vi "experiment_med_read_FF.vi"() -> ()   [LabVIEW 2018]
uses:
  FPGA/Feed forward/FeedForwardState.ctl
  <vilib>/rvi/Emulation/niFpgaSctlEmulationGetInTimedLoop.vi
  <vilib>/rvi/Memory/Memory_Emulation/nirvimemoryFastEmulation.vi
  <vilib>/rvi/Memory/Memory_Emulation/nirvimemoryEmulation.vi
  <vilib>/rvi/Emulation/niFpgaEmulationIsFPGAContextNoSignature.vi
  <vilib>/rvi/DataTransferAndStorage/Container/Common/niFpgaContainerGetUniqueNameForEmu.vi
  <vilib>/rvi/Emulation/niFpgaProcessEmulError.vi
  <vilib>/rvi/errors/nirviReportUnexpectedCaseInternalError (U32).vi
  <instrlib>/_niInstr/Basic Elements/v1/FPGA/Private/Count Down U8.vi
  <vilib>/rvi/DataTransferAndStorage/Container/XNode/niFpgaContainer.xnode
  <instrlib>/_niInstr/Basic Elements/v1/FPGA/niInstr Basic Elements v1 FPGA.lvlib
panel:
  out "Array":dbl[](array[numeric])
  out "Waveform Graph":dbl[](graph)
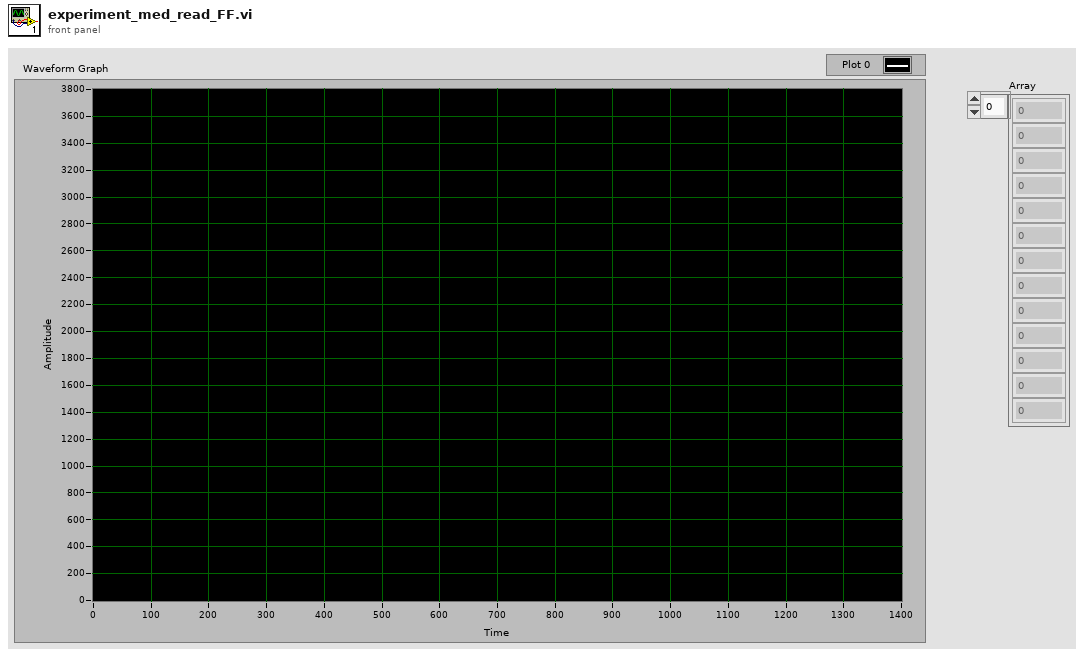
[diagram p1: front panel]
types:
  T1 = typedef "FeedForwardState.ctl" = enum16{"Idle", "Wait for trigger", "Read FF", "Clear FF", "Wait for reset"}
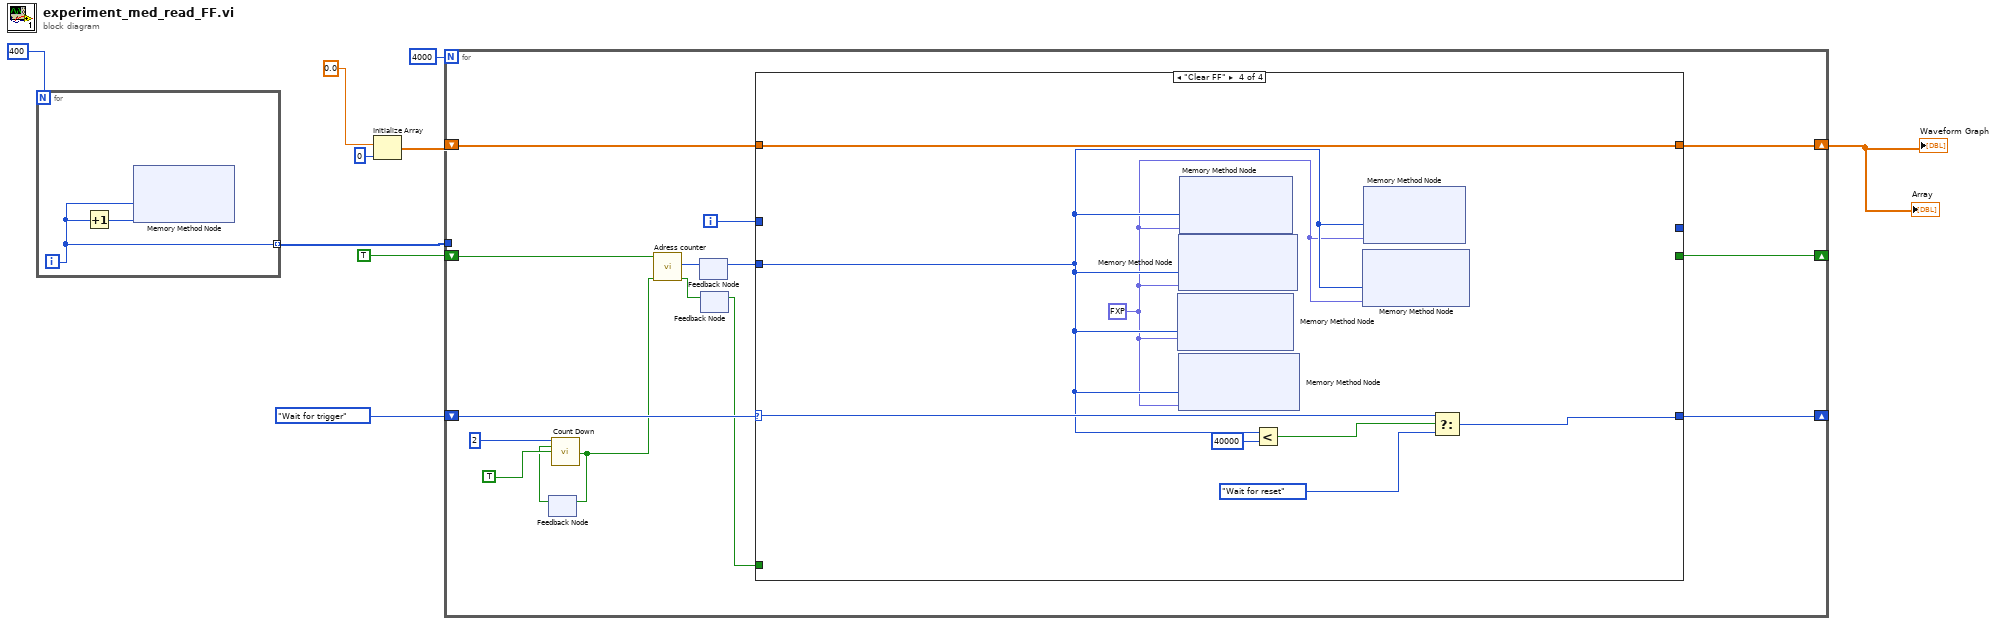
[diagram p0: block diagram]
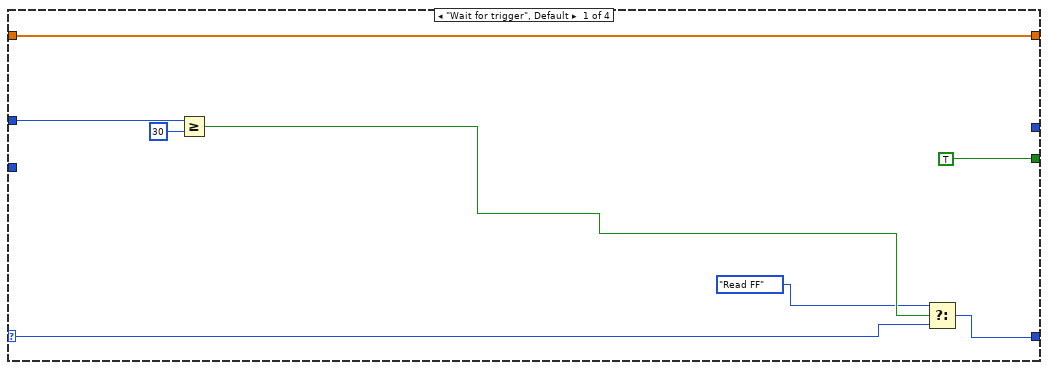
[diagram p2: hidden frame]
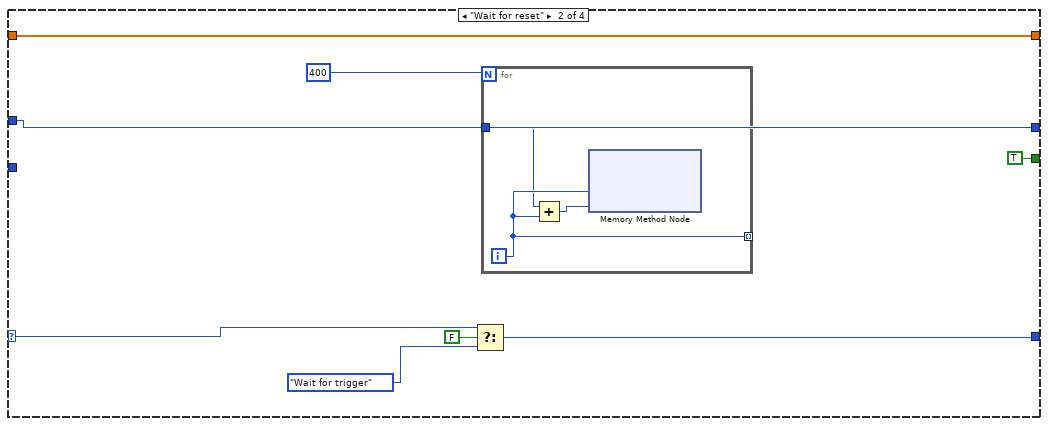
[diagram p3: hidden frame]
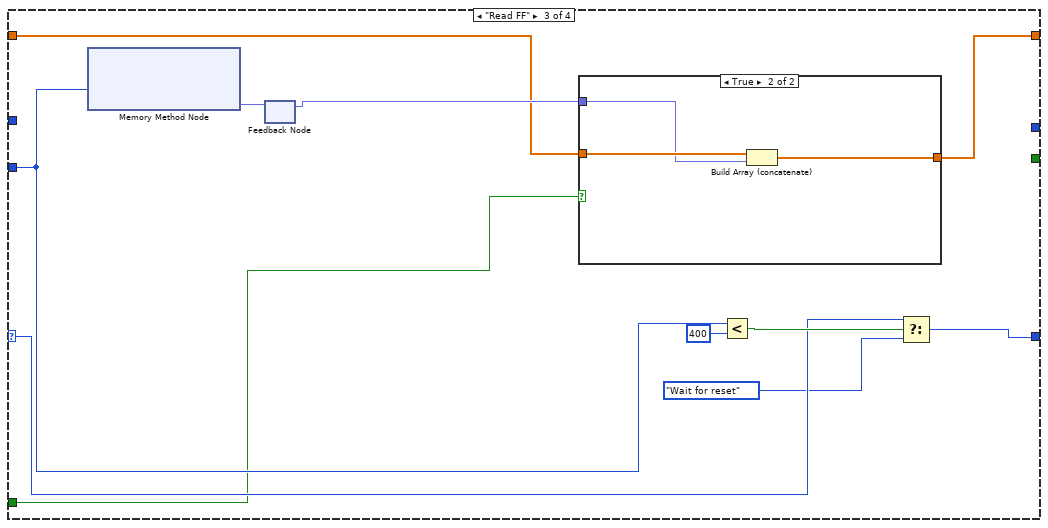
[diagram p4: hidden frame]
diagram:
  n1 = for {
    N: 400 -> [_]
    tunnel: [w10] -> w5 mode=indexing
    i -> [w10]
    n2 = Increment(x=w10) -> (x+1=w11:i32)
    n3 = xnode ("Memory Method Node")("Address"=w10, "Data"=w11) -> ()  [unwired: 1 in, 1 out]
  }
  n4 = Initialize Array(0.0, 0 ("dimension size")) -> (w2:dbl[])
  n5 = for {
    N: 4000 -> [_]
    shift-right: [w17] -> _
    shift-left: FeedForwardState."Wait for trigger" ("FF state") -> [w24]
    shift-right: [w18] -> _
    shift-left: TRUE ("decrement") -> [w19]
    tunnel: w5 -> [_]
    shift-right: [w14] -> w1
    shift-left: w2 -> [w15]
    i -> [w16]
    n6 = feedback #1() -> (w21:bool)  [unwired: 1 in]
    n7 = call-poly <instrlib>:"Count Down.vi"("count in"=u8 2, "load"=w21, "decrement"=TRUE) -> ("terminal count"=w20:bool)  [unwired: 11 in, 1 out]
    n8 = feedback-in #1(w20) -> ()
    n9 = call "Adress counter.vi"("input valid"=w20, "Reset"=w19) -> ("output valid"=w13:bool, "Address"=w26:u32)  [unwired: 8 in]
    n10 = feedback #2() -> (w25:u32)  [unwired: 1 in]
    n11 = feedback-in #2(w26) -> ()
    n12 = feedback #3() -> (w12:bool)  [unwired: 1 in]
    n13 = feedback-in #3(w13) -> ()
    n14 = case shown="\"Clear FF\"" w24 {
      selector: w24 -> [w33 w39 w54 w65]
      tunnel: w25 -> [_ _ w51 w63]
      tunnel: [w32 w42 w53 w64] -> w17
      tunnel: w12 -> [_ _ w46 _]
      tunnel: [TRUE ("decrement") TRUE ("decrement") _ _] -> w18
      tunnel: w16 -> [w31 w35 _ _]
      tunnel: w15 -> [w27 w37 w48 w61]
      tunnel: [w27 w37 w47 w61] -> w14
      tunnel: [_ w35 _ _] -> _
      frame "Wait for trigger", Default {
        n15 = Greater Or Equal?(x=w31, y=30) -> (x >= y?=w29:bool)
        n16 = Select(t=FeedForwardState."Read FF" ("FF state"), s=w29, f=w33) -> (s? t:f=w32:T1)
      }
      frame "Wait for reset" {
        n17 = Select(t=w39, s=FALSE, f=FeedForwardState."Wait for trigger" ("FF state")) -> (s? t:f=w42:T1)
        n18 = for {
          N: 400 -> [_]
          tunnel: [w45] -> _ mode=indexing
          tunnel: w35 -> [w44]
          i -> [w45]
          n19 = Add(x=w44, y=w45) -> (x+y=w43:i32)
          n20 = xnode ("Memory Method Node")("Address"=w45, "Data"=w43) -> ()  [unwired: 1 in, 1 out]
        }
      }
      frame "Read FF" {
        n21 = xnode ("Memory Method Node")("Address"=w51) -> ("Data"=w50:fxp<+/-,32,14>)  [unwired: 1 in, 1 out]
        n22 = feedback #4() -> (w49:fxp<+/-,32,14>)  [unwired: 1 in]
        n23 = feedback-in #4(w50) -> ()
        n24 = case shown="True" w46 {
          tunnel: w49 -> [_ w59]
          tunnel: w48 -> [w57 w60]
          tunnel: [w57 w58] -> w47
          frame False {
          }
          frame True {
            n25 = Build Array (concatenate)(w60, w59) -> (w58:dbl[])
          }
        }
        n26 = Less?(x=w51, y=u32 400) -> (x < y?=w55:bool)
        n27 = Select(t=w54, s=w55, f=FeedForwardState."Wait for reset" ("FF state")) -> (s? t:f=w53:T1)
      }
      frame "Clear FF" {
        w62 = fxp<+/-,32,14> 0.0 ("Data")
        n28 = xnode ("Memory Method Node")("Address"=w63, "Data"=w62) -> ()  [unwired: 1 in, 1 out]
        n29 = xnode ("Memory Method Node")("Address"=w63, "Data"=w62) -> ()  [unwired: 1 in, 1 out]
        n30 = xnode ("Memory Method Node")("Address"=w63, "Data"=w62) -> ()  [unwired: 1 in, 1 out]
        n31 = xnode ("Memory Method Node")("Address"=w63, "Data"=w62) -> ()  [unwired: 1 in, 1 out]
        n32 = Less?(x=w63, y=u32 40000) -> (x < y?=w67:bool)
        n33 = xnode ("Memory Method Node")("Address"=w63, "Data"=w62) -> ()  [unwired: 1 in, 1 out]
        n34 = xnode ("Memory Method Node")("Address"=w63, "Data"=w62) -> ()  [unwired: 1 in, 1 out]
        n35 = Select(t=w65, s=w67, f=FeedForwardState."Wait for reset" ("FF state")) -> (s? t:f=w64:T1)
      }
    }
  }
  "Waveform Graph" <- w1
  "Array" <- w1
